vi "ma_Compute t0 eps DBL.vi"(10 "t0 entry":dbl format="%0.6e") -> (3 "t0 eps":dbl format="%0.6e")   [LabVIEW 2020, in "NI_MABase.lvlib"]
uses:
  NI_MABase.lvlib
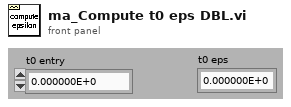
[diagram p1: front panel]
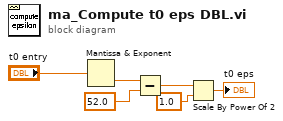
[diagram p0: block diagram]
diagram:
  n1 = Mantissa & Exponent(0:"t0 entry") -> (2:w4:dbl)  [unwired: 1 out]
  n2 = Subtract(x=w4, y=52.0 ("x")) -> (x-y=w6:dbl)
  n3 = Scale By Power Of 2(n=w6, x=1.0) -> (x*2^n=→"t0 eps":dbl)
